vi "onGetResultsName.vi"(8 "error in (no error)":errorcluster, 11 "Pips.TestResults in":refnum<class "Pips.TestResults.lvclass">) -> (0 "error out":errorcluster, 2 "Name":string, 3 "Pips.TestResults out":refnum<class "Pips.TestResults.lvclass">)   [LabVIEW 2021, in "Banana.Caraya.lvlib" / "Pips.TestResults.lvclass"]
uses:
  Pips.TestResults.lvclass
  Pips.TestResults.lvclass/Pips.TestResults.ctl
  <vilib>/addons/_JKI Toolkits/Caraya/classes/Test Result/Test Result.lvclass
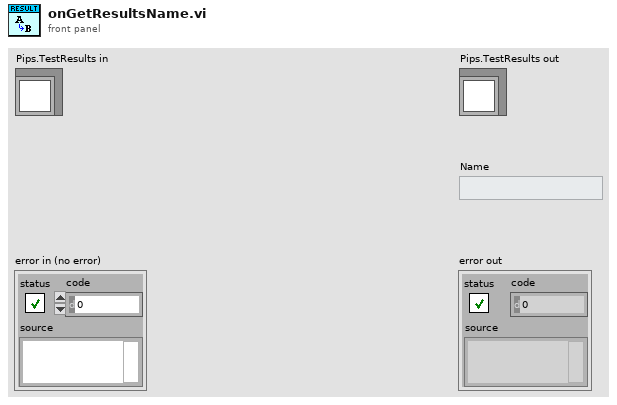
[diagram p1: front panel]
types:
  T1 = typedef "Caraya.lvlib/Test Result.lvclass/Test Node (Extended).ctl" = cluster{"Test Registration":T2, "Defined":bool, "Passed":bool, "properties":variant}
  T2 = typedef "Caraya.lvlib/Test Result.lvclass/Test Registration Data.ctl" = cluster{"Name":string, "Call Chain":string[], "Time Stamp":timestamp, "Test ID":string, "Caller ID":string}
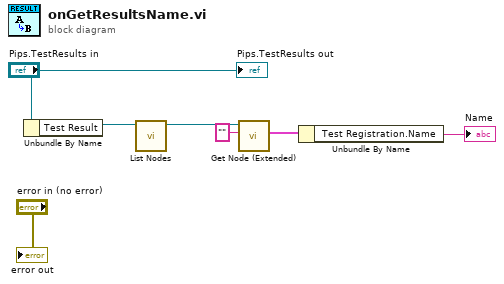
[diagram p0: block diagram]
diagram:
  n1 = Unbundle By Name("Pips.TestResults in") -> ("Test Result"=w5:refnum<class "Test Result.lvclass">)
  n2 = call <vilib>:"List Nodes.vi"("Test Result in"=w5) -> ("Test Result out"=w4:refnum<class "Test Result.lvclass">)  [unwired: 8 in, 2 out]
  n3 = call <vilib>:"Get Node (Extended).vi"("Node"="", "Test Result in"=w4) -> ("Test Node"=w2:T1)  [unwired: 4 in, 5 out]
  n4 = Unbundle By Name(w2) -> ("Test Registration.Name"=→"Name":string)
  "error out" <- "error in (no error)"
  "Pips.TestResults out" <- "Pips.TestResults in"
